vi "lab 1.1.vi"() -> ()   [LabVIEW 2021]
uses:
  <vilib>/express/express analysis/Spectral/Block/exnSpectralBlock spectral measurements peak poly.vi
  <vilib>/express/express analysis/Spectral/Block/exnSpectralBlock spectral measurements peak DDT.vi
  <vilib>/express/express analysis/Spectral/XNode/ExpressSpectralMeasurementsBlockNode.xnode
panel:
  out "Waveform Graph hanning":dynamicdata(graph)
  out "Waveform Graph Rectangular":dynamicdata(graph)
  out "Waveform Graph":dynamicdata(graph)
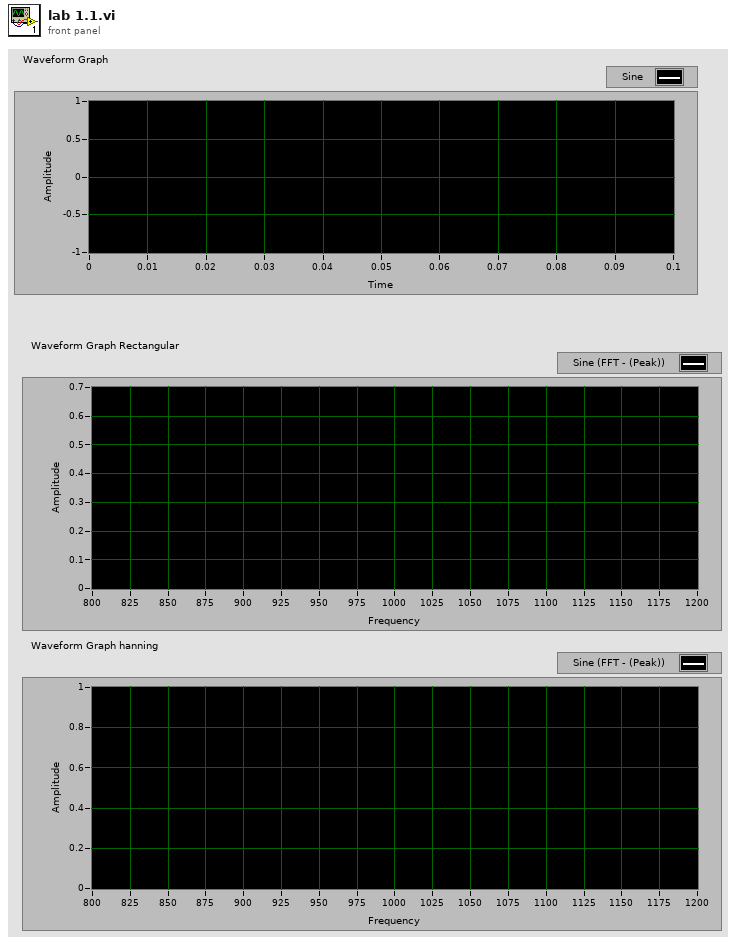
[diagram p1: front panel]
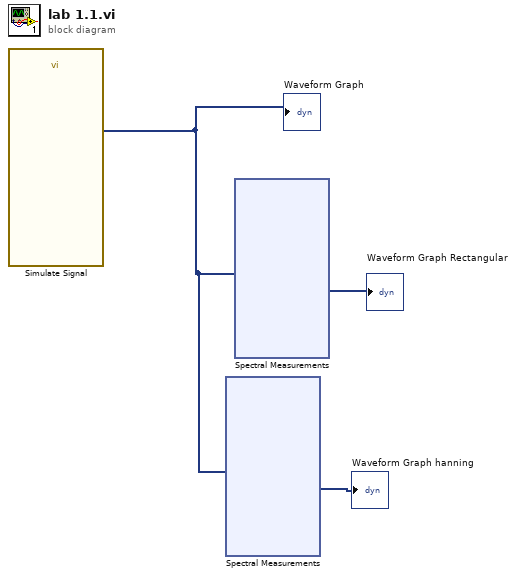
[diagram p0: block diagram]
diagram:
  n1 = call "Simulate Signal"() -> ("Sine"=w1:dynamicdata)  [unwired: 14 in, 1 out]
  "Waveform Graph" <- w1
  n2 = xnode "Spectral Measurements"("Signals"=w1) -> ("FFT - (Peak)"=→"Waveform Graph hanning":dynamicdata)  [unwired: 1 in, 2 out]
  n3 = xnode "Spectral Measurements"("Signals"=w1) -> ("FFT - (Peak)"=→"Waveform Graph Rectangular":dynamicdata)  [unwired: 1 in, 2 out]
